vi "send.vi"(8 "error in (no error)":errorcluster, 10 "messge":string, 11 "TCP_IP (in)":refnum<class "TCP_IP.lvclass">) -> (0 "error out":errorcluster)   [LabVIEW 2013, in "TCP_IP.lvclass"]
uses:
  TCP_IP.lvclass
  TCP_IP.lvclass/TCP_IP.ctl
  Globals.vi
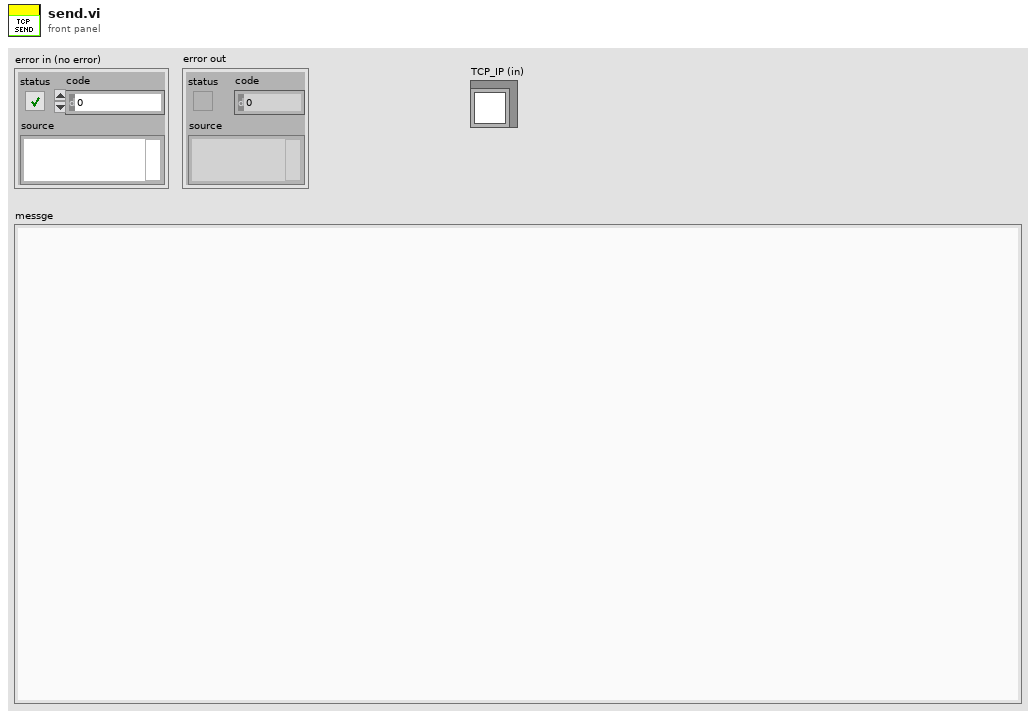
[diagram p1: front panel]
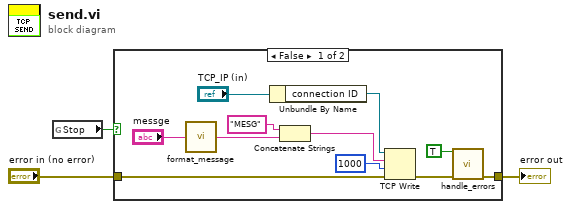
[diagram p0: block diagram]
diagram:
  n1 = global read "Globals.vi" "Stop"() -> (w1:bool)
  n2 = case shown="False" w1 {
    tunnel: [w12 w15] -> w3
    tunnel: "error in (no error)" -> [w11 w15]
    frame False {
      n3 = call "format_message.vi"("messge"="messge") -> ("concatenated string"=w6:string)
      n4 = Unbundle By Name("TCP_IP (in)") -> ("connection ID"=w8:refnum<k5>)
      n5 = Concatenate Strings("MESG", w6) -> (w5:string)
      n6 = TCP Write(connection ID=w8, data in=w5, error in (no error)=w11, 9:1000 ("timeout ms (25000)")) -> (error out=w13:errorcluster)  [unwired: 2 out]
      n7 = call "handle_errors.vi"("Exit Operation"=TRUE ("Exit Measurement"), "error in (no error)"=w13) -> ("error out"=w12:errorcluster)  [unwired: 13 in]
    }
    frame True {
    }
  }
  "error out" <- w3
